vi "digital to decimal.vi"() -> ()   [LabVIEW 2012]
panel:
  in  "Array 2":dbl[][](array[numeric])
  out "Array":dbl[](array[numeric])
  out "Numeric 2":i32
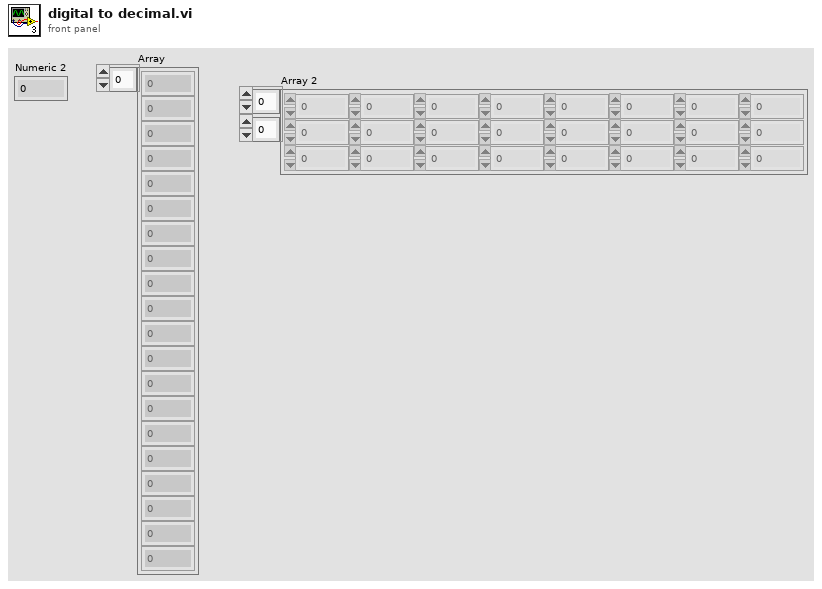
[diagram p1: front panel]
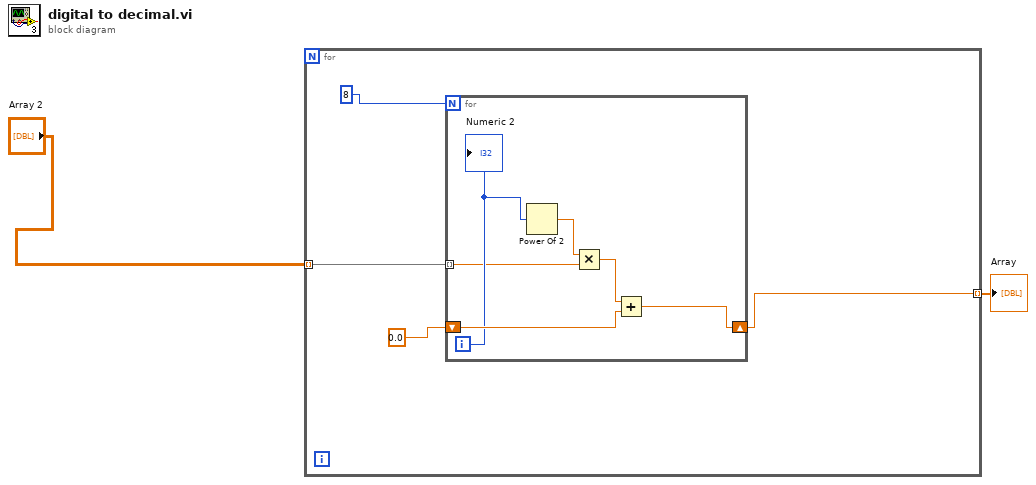
[diagram p0: block diagram]
diagram:
  n1 = for {
    tunnel: [w4] -> w2 mode=indexing
    tunnel: "Array 2" -> [w3] mode=indexing
    n2 = for {
      N: 8 -> [_]
      shift-right: [w10] -> w4
      shift-left: 0.0 -> [w11]
      tunnel: w3 -> [w7] mode=indexing
      i -> [w9]
      n3 = Power Of 2(x=w9) -> (2^x=w8:dbl)
      n4 = Multiply(x=w8, y=w7) -> (x*y=w12:dbl)
      n5 = Add(x=w12, y=w11) -> (x+y=w10:dbl)
      "Numeric 2" <- w9
    }
  }
  "Array" <- w2
